vi "SWPS.vi"() -> ()   [LabVIEW 2020]
panel:
  in  "L1":dbl
  in  "Mz":dbl
  in  "J":dbl step=0.1
  in  "Menu Ring":u16(ring) items=["Home", "Stan ustalony   Sterowanie Twornikowe   Charakterystyka regulacyjna", "Stan ustalony   Sterowanie Twornikowe   Charakterystyka mechaniczna", "Stan ustalony   Sterowanie Biegunowe   Charakterystyka regulacyjna", "Stan ustalony   Sterowanie Biegunowe   Charakterystyka mechaniczna", "Stan nieustalony   Sterowanie Twornikowe", "Stan nieustalony   Sterowanie Biegunowe"]
  out "Waveform Graph":waveform(dbl)(graph)
  in  "Me":dbl=1.0 step=0.1
  in  "Lm":dbl=2.0
  in  "R2":dbl=50.0
  in  "R1":dbl=400.0
  in  "U2":dbl=25.0
  in  "U1":dbl=100.0
  in  "Home Button":bool
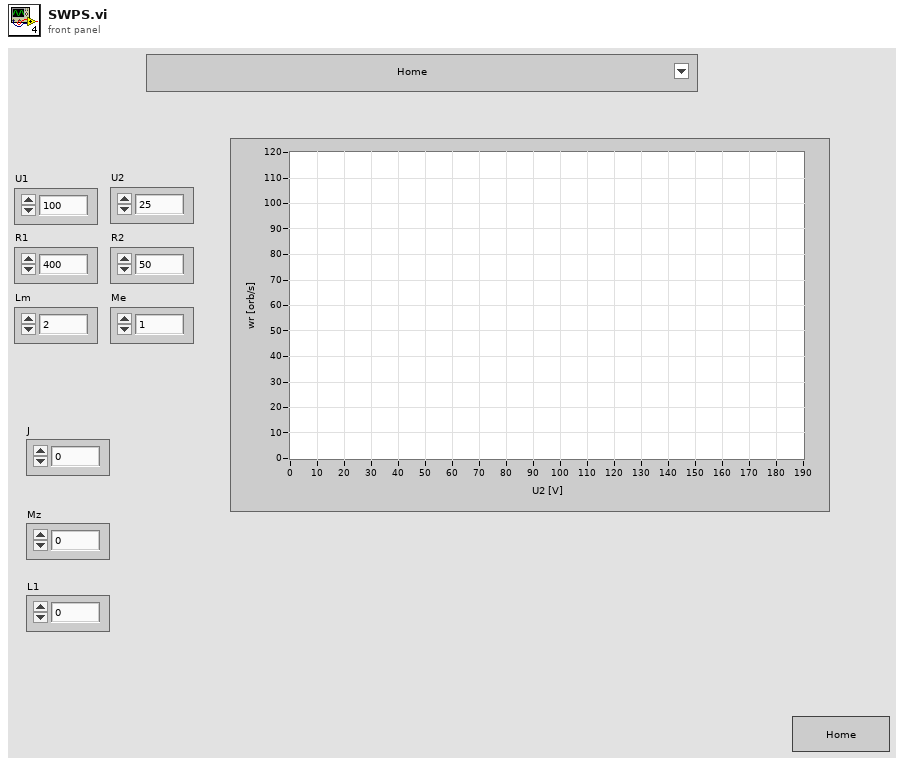
[diagram p1: front panel]
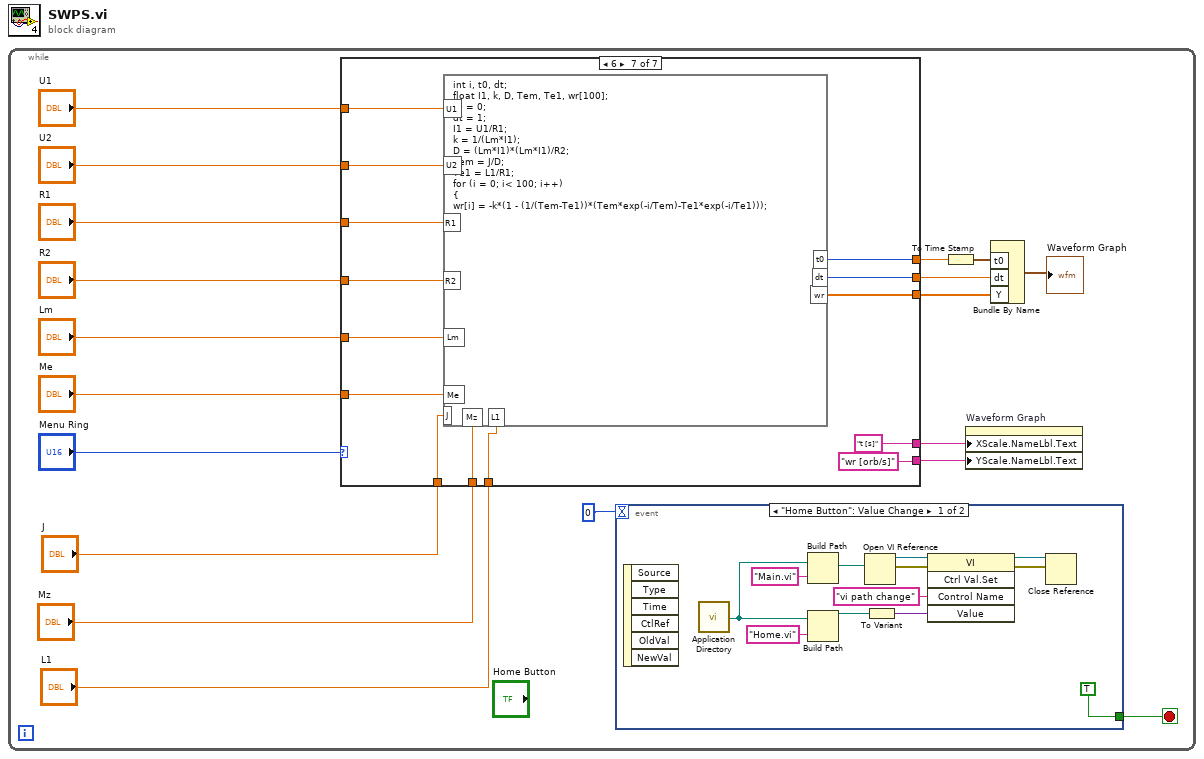
[diagram p0: block diagram]
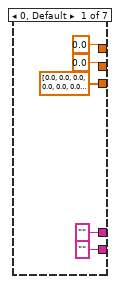
[diagram p2: hidden frame]
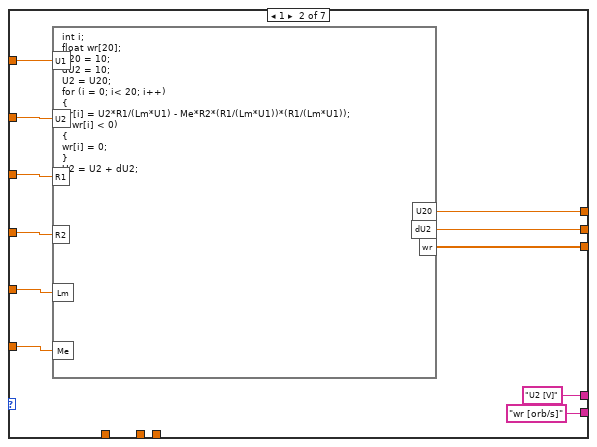
[diagram p3: hidden frame]
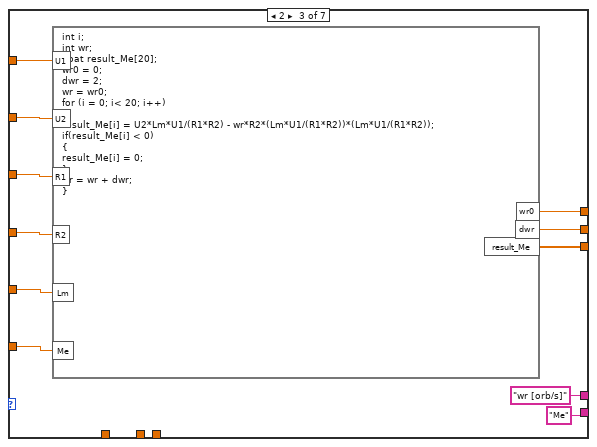
[diagram p4: hidden frame]
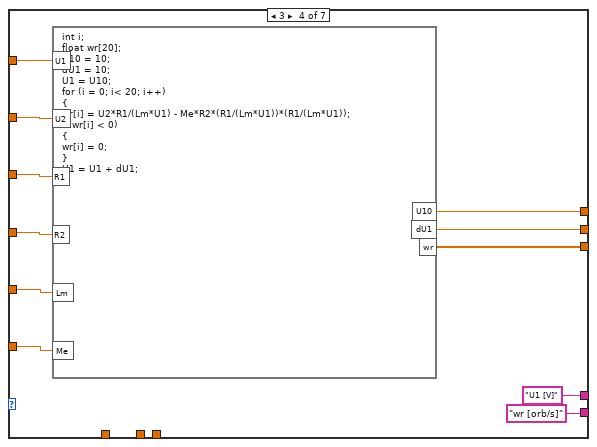
[diagram p5: hidden frame]
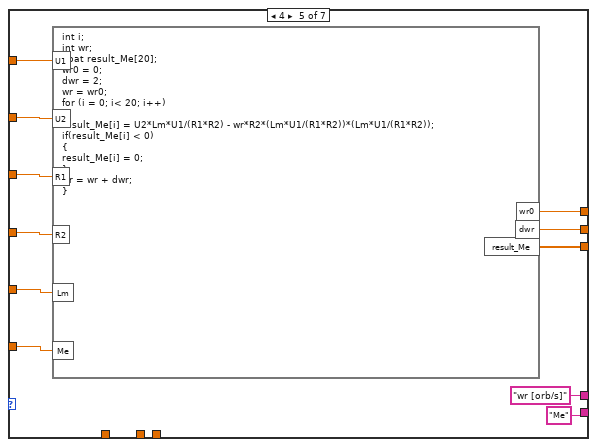
[diagram p6: hidden frame]
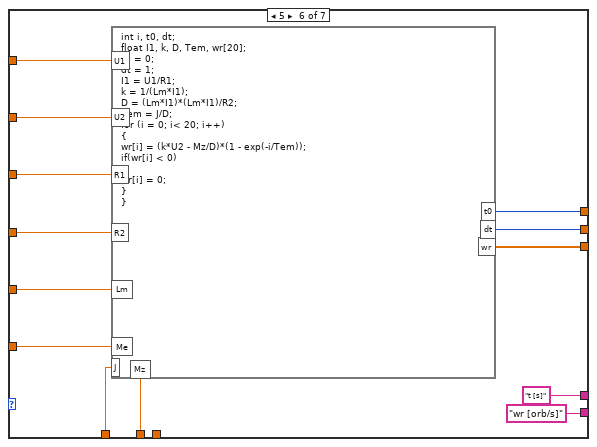
[diagram p7: hidden frame]
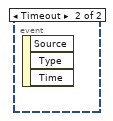
[diagram p8: hidden frame]
diagram:
  n1 = while {
    stop <- w8 stop-if-true
    n2 = case shown="6" "Menu Ring" {
      tunnel: "U1" -> [_ w35 w46 w57 w68 w81 w95]
      tunnel: "U2" -> [_ w34 w45 w56 w67 w80 w94]
      tunnel: "R1" -> [_ w33 w44 w55 w66 w79 w93]
      tunnel: "R2" -> [_ w32 w43 w54 w65 w78 w92]
      tunnel: "Lm" -> [_ w31 w42 w53 w64 w77 w91]
      tunnel: "Me" -> [_ w30 w41 w52 w63 w76 w90]
      tunnel: [dbl[] [0.0, 0.0, 0.0, 0.0, 0.0, 0.0, 0.0, 0.0, 0.0, 0.0, 0.0, 0.0, 0.0, 0.0, 0.0, 0.0, 0.0, 0.0, 0.0, 0.0] w29 w38 w51 w60 w75 w89] -> w13
      tunnel: [0.0 ("dwr") w28 w40 w47 w62 w74 w88] -> w12
      tunnel: [0.0 ("wr0") w27 w39 w50 w61 w73 w87] -> w10
      tunnel: ["" "U2 [V]" "wr [orb/s]" "U1 [V]" "wr [orb/s]" "t [s]" "t [s]"] -> w5
      tunnel: ["" "wr [orb/s]" "Me" "wr [orb/s]" "Me" "wr [orb/s]" "wr [orb/s]"] -> w4
      tunnel: "J" -> [_ _ _ _ _ w70 w84]
      tunnel: "Mz" -> [_ _ _ _ _ w69 w83]
      tunnel: "L1" -> [_ _ _ _ _ _ w82]
      frame 0, Default {
      }
      frame 1 {
        n3 = formula code="int i;\nfloat wr[20];\nU20 = 10;\ndU2 = 10;\nU2 = U20;\nfor (i = 0; i< 20; i++)\n{\nwr[i] = U2*R1/(Lm*U1) - Me*R2*(R1/(Lm*U1))*(R1/(Lm*U1));\nif(wr[i] < 0)\n{\nwr[i] = 0;\n}\nU2 = U2 + dU2;\n}"("U1"=w35, "U2"=w34, "R1"=w33, "R2"=w32, "Lm"=w31, "Me"=w30) -> ("wr"=w29:dbl[], "dU2"=w28:dbl, "U20"=w27:dbl)
      }
      frame 2 {
        n4 = formula code="int i;\nint wr;\nfloat result_Me[20];\nwr0 = 0;\ndwr = 2;\nwr = wr0;\nfor (i = 0; i< 20; i++)\n{\nresult_Me[i] = U2*Lm*U1/(R1*R2) - wr*R2*(Lm*U1/(R1*R2))*(Lm*U1/(R1*R2));\nif(result_Me[i] < 0)\n{\nresult_Me[i] = 0;\n}\nwr = wr + dwr;\n}"("U1"=w46, "U2"=w45, "R1"=w44, "R2"=w43, "Lm"=w42, "Me"=w41) -> ("result_Me"=w38:dbl[], "dwr"=w40:dbl, "wr0"=w39:dbl)
      }
      frame 3 {
        n5 = formula code="int i;\nfloat wr[20];\nU10 = 10;\ndU1 = 10;\nU1 = U10;\nfor (i = 0; i< 20; i++)\n{\nwr[i] = U2*R1/(Lm*U1) - Me*R2*(R1/(Lm*U1))*(R1/(Lm*U1));\nif(wr[i] < 0)\n{\nwr[i] = 0;\n}\nU1 = U1 + dU1;\n}"("U1"=w57, "U2"=w56, "R1"=w55, "R2"=w54, "Lm"=w53, "Me"=w52) -> ("wr"=w51:dbl[], "dU1"=w47:dbl, "U10"=w50:dbl)
      }
      frame 4 {
        n6 = formula code="int i;\nint wr;\nfloat result_Me[20];\nwr0 = 0;\ndwr = 2;\nwr = wr0;\nfor (i = 0; i< 20; i++)\n{\nresult_Me[i] = U2*Lm*U1/(R1*R2) - wr*R2*(Lm*U1/(R1*R2))*(Lm*U1/(R1*R2));\nif(result_Me[i] < 0)\n{\nresult_Me[i] = 0;\n}\nwr = wr + dwr;\n}"("U1"=w68, "U2"=w67, "R1"=w66, "R2"=w65, "Lm"=w64, "Me"=w63) -> ("result_Me"=w60:dbl[], "dwr"=w62:dbl, "wr0"=w61:dbl)
      }
      frame 5 {
        n7 = formula code="int i, t0, dt;\nfloat I1, k, D, Tem, wr[20];\nt0 = 0;\ndt = 1;\nI1 = U1/R1;\nk = 1/(Lm*I1);\nD = (Lm*I1)*(Lm*I1)/R2;\nTem = J/D;\nfor (i = 0; i< 20; i++)\n{\nwr[i] = (k*U2 - Mz/D)*(1 - exp(-i/Tem));\nif(wr[i] < 0)\n{\nwr[i] = 0;\n}\n}"("U1"=w81, "U2"=w80, "R1"=w79, "R2"=w78, "Lm"=w77, "Me"=w76, "J"=w70, "Mz"=w69) -> ("wr"=w75:dbl[], "dt"=w74:i32, "t0"=w73:i32)
      }
      frame 6 {
        n8 = formula code="int i, t0, dt;\nfloat I1, k, D, Tem, Te1, wr[100];\nt0 = 0;\ndt = 1;\nI1 = U1/R1;\nk = 1/(Lm*I1);\nD = (Lm*I1)*(Lm*I1)/R2;\nTem = J/D;\nTe1 = L1/R1;\nfor (i = 0; i< 100; i++)\n{\nwr[i] = -k*(1 - (1/(Tem-Te1))*(Tem*exp(-i/Tem)-Te1*exp(-i/Te1)));\n}"("U1"=w95, "U2"=w94, "R1"=w93, "R2"=w92, "Lm"=w91, "Me"=w90, "J"=w84, "Mz"=w83, "L1"=w82) -> ("wr"=w89:dbl[], "dt"=w88:i32, "t0"=w87:i32)
      }
    }
    n9 = event shown="[0] \"Home Button\": Value Change" {
      selector: _ -> [_ _]
      dyn-events: _ -> [_ _]
      timeout: 0 -> [_ _]
      tunnel: [TRUE _] -> w8
      event "Home Button": Value Change {
        n10 = event-data() -> ()  [unwired: 1 in, 6 out]
        n11 = call <vilib>:"Application Directory.vi"() -> ("Application Directory"=w97:path)
        n12 = Build Path(base path=w97, name or relative path="Main.vi") -> (appended path=w98:path)
        n13 = Build Path(base path=w97, name or relative path="Home.vi") -> (appended path=w100:path)
        n14 = Open VI Reference(vi path=w98) -> (vi reference=w105:refnum<vi>, error out=w106:errorcluster)  [unwired: 5 in]
        n15 = To Variant(anything=w100) -> (Variant=w107:variant)
        n16 = invoke class="VI" method="Ctrl Val.Set"(reference=w105, error in=w106, "Control Name"="vi path change", "Value"=w107) -> (reference out=w104:refnum<vi>, error out=w103:errorcluster)  [unwired: 1 in, 3 out]
        n17 = Close Reference(reference=w104, error in (no error)=w103) -> ()  [unwired: 1 out]
      }
      event Timeout {
        n18 = event-data() -> ()  [unwired: 1 in, 3 out]
      }
    }
    n19 = To Time Stamp(1:w10) -> (0:w11:timestamp)
    n20 = property on="Waveform Graph" class="WFGraph (strict)"("XScale.NameLbl.Text"=w5, "YScale.NameLbl.Text"=w4) -> ()  [unwired: 2 in, 2 out]
    n21 = Bundle By Name("t0"=w11, "dt"=w12, "Y"=w13) -> (→"Waveform Graph":waveform(dbl))  [unwired: 1 in]
  }
